vi "Solenoid Get.vi"(10 "DevRef":string) -> (0 "Error Out":errorcluster, 3 "PneumaticsDevRefOut":T1={"Pneumatic State Reference"=refnum, "SolenoidDevRef"={"DevStatus"={"status"=FALSE, "code"=0, "source"=""}, "Pneumatics Control Module"=0, "Forward Solenoid Channel"=enum."Invalid", "Reverse Solenoid Channel"=enum."Invalid"}, "Pneumatic Configuration reference"=refnum})   [LabVIEW 2015]
uses:
  <userlib>/836-Library/Pneumatics/Pneumatics/836_PneumaticsDevRef.ctl
  <userlib>/836-Library/Pneumatics/Pneumatics/Pneumatic State.ctl
  <userlib>/836-Library/Pneumatics/Pneumatics/StateMachine.ctl
  <vilib>/Rock Robotics/WPI/Solenoid/WPI_SolenoidDevRef.ctl
  <vilib>/Rock Robotics/WPI/Solenoid/WPI_SolenoidChannel.ctl
  <userlib>/836-Library/Pneumatics/Pneumatics/Pneumatic Configuration.ctl
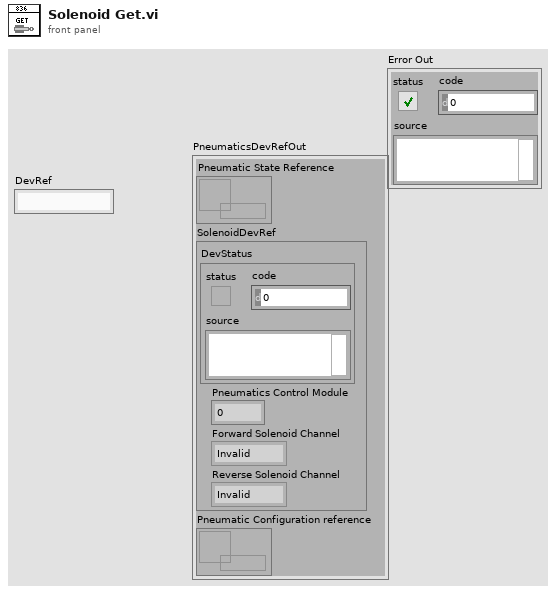
[diagram p1: front panel]
types:
  T1 = typedef "836_PneumaticsDevRef.ctl" = cluster{"Pneumatic State Reference":refnum<data-value>, "SolenoidDevRef":T2, "Pneumatic Configuration reference":refnum<data-value>}
  T2 = typedef "WPI_SolenoidDevRef.ctl" = cluster{"DevStatus":errorcluster, "Pneumatics Control Module":u8, "Forward Solenoid Channel":T3, "Reverse Solenoid Channel":T3}
  T3 = typedef "WPI_SolenoidChannel.ctl" = enum8{"Solenoid 0", "Solenoid 1", "Solenoid 2", "Solenoid 3", "Solenoid 4", "Solenoid 5", "Solenoid 6", "Solenoid 7", "Invalid"}
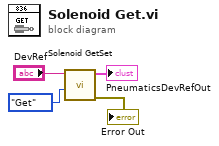
[diagram p0: block diagram]
diagram:
  n1 = call <userlib>:"Solenoid GetSet.vi"("Enum"=enum16{"Set", "Get"}."Get", "DevRef"="DevRef") -> ("Error Out"=→"Error Out":errorcluster, "PneumaticsDevRef out"=→"PneumaticsDevRefOut":T1)  [unwired: 8 in]
